vi "Write Is Connected.vi"(8 "error in (no error)":errorcluster, 10 "Connected?":bool, 11 "WAMP Client in":refnum<class "WAMP Client.lvclass">) -> (0 "error out":errorcluster, 3 "WAMP Client out":refnum<class "WAMP Client.lvclass">)   [LabVIEW 2021, in "wamplv.lvlib" / "WAMP Client.lvclass"]
uses:
  WAMP Client.lvclass
  WAMP Client.lvclass/WAMP Client.ctl
  API/TypeDefs/Disconnected event data.ctl
  TypeDef/Termination Reason.ctl
  TypeDef/Termination Reason Enum.ctl
  API/TypeDefs/Connected event data.ctl
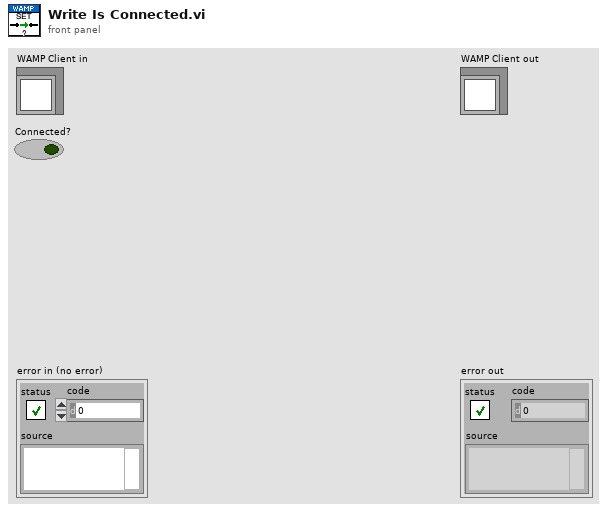
[diagram p1: front panel]
types:
  T1 = typedef "wamplv.lvlib/WAMP Client.lvclass/Disconnected event data.ctl" = cluster{"Error Out":errorcluster, "Termination Reason":T2}
  T2 = typedef "wamplv.lvlib/WAMP Client.lvclass/Termination Reason.ctl" = cluster{"Reason":T3, "Reason URI":string, "Message":string}
  T3 = typedef "wamplv.lvlib/WAMP Client.lvclass/Termination Reason Enum.ctl" = enum16{"Goodbye Received", "Abort Received", "Send Goodbye", "Send Abort", "Read Loop Failure", "Write Loop Failure", "Message Loop Failure"}
  T4 = typedef "wamplv.lvlib/WAMP Client.lvclass/Connected event data.ctl" = cluster{"Session ID":u64}
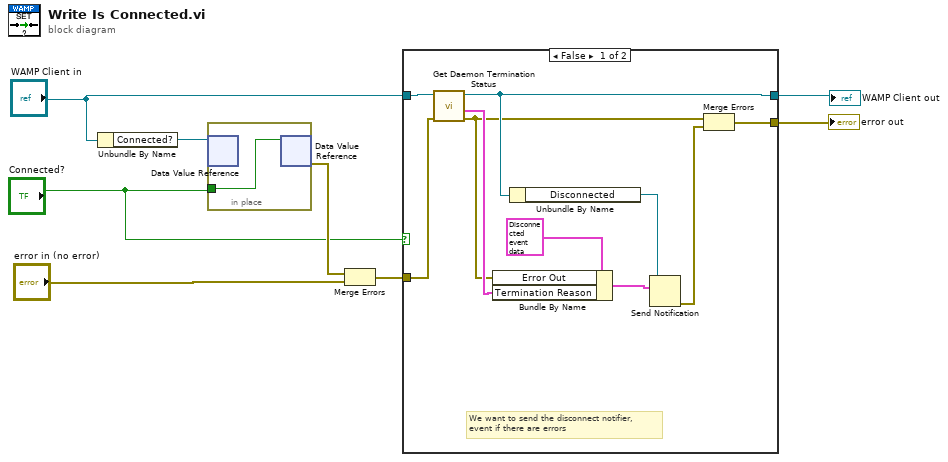
[diagram p0: block diagram]
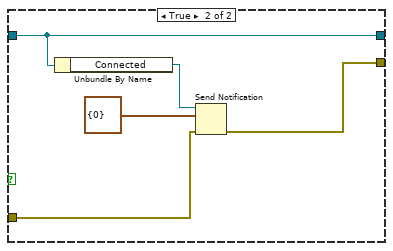
[diagram p2: hidden frame]
diagram:
  n1 = Unbundle By Name("WAMP Client in") -> ("Connected?"=w7:refnum<data-value>)
  n2 = in-place {
    in-place-border: "Connected?" -> [w9]
    n3 = in-place-dvr #1(w7) -> ()  [unwired: 2 out]
    n4 = in-place-dvr #1(w9) -> (w6:errorcluster)  [unwired: 1 out]
  }
  n5 = Merge Errors(w6, "error in (no error)") -> (w1:errorcluster)
  n6 = case shown="False" "Connected?" {
    tunnel: "WAMP Client in" -> [w19 w24]
    tunnel: [w14 w24] -> w3
    tunnel: [w12 w22] -> w2
    tunnel: w1 -> [w17 w21]
    frame False {
      # "We want to send the disconnect notifier,\nevent if there are errors"
      n7 = call "Get Daemon Termination Status.vi"("error in (no error)"=w17, "WAMP Client in"=w19) -> ("error out"=w11:errorcluster, "Termination Reason"=w15:T2, "WAMP Client out"=w14:refnum<class "WAMP Client.lvclass">)  [unwired: 6 in, 1 out]
      n8 = Bundle By Name(cluster=T1 {"Error Out"={"status"=FALSE, "code"=0, "source"=""}, "Termination Reason"={"Reason"=enum."Goodbye Received", "Reason URI"="wamp.error.protocol_violation", "Message"=""}} ("Cluster"), "Error Out"=w11, "Termination Reason"=w15) -> (w13:T1)
      n9 = Unbundle By Name(w14) -> ("Disconnected"=w16:refnum<notifier>)
      n10 = Send Notification(notification=w13, notifier=w16) -> (error out=w10:errorcluster)  [unwired: 1 in, 1 out]
      n11 = Merge Errors(w11, w10) -> (w12:errorcluster)
    }
    frame True {
      n12 = Unbundle By Name(w24) -> ("Connected"=w23:refnum<notifier>)
      n13 = Send Notification(notification=T4 {"Session ID"=0} ("Connected event data"), notifier=w23, error in (no error)=w21) -> (error out=w22:errorcluster)  [unwired: 1 out]
    }
  }
  "error out" <- w2
  "WAMP Client out" <- w3
